vi "FL_Save_incrementally_ts.vi"(0 "Temporary file output path":path, 1 "Play / Pause":bool, 2 "Sensor read input":sgl[][](array[numeric]), 5 "Loop iteration":i32, 7 "Loop speed in ms":u16, 9 "Save every N seconds":u32=15, 11 "error in (no error)":errorcluster, 12 "Current_Time":timestamp, 13 "Start_Time":timestamp) -> (4 "Eff. save interval":sgl, 15 "error out":errorcluster)   [LabVIEW 2018, in "Tracker.lvlib"]
uses:
  Tracker.lvlib
  <vilib>/Utility/file.llb/Write Delimited Spreadsheet (DBL).vi
panel:
  out "transposed array":dbl[][](array[numeric])
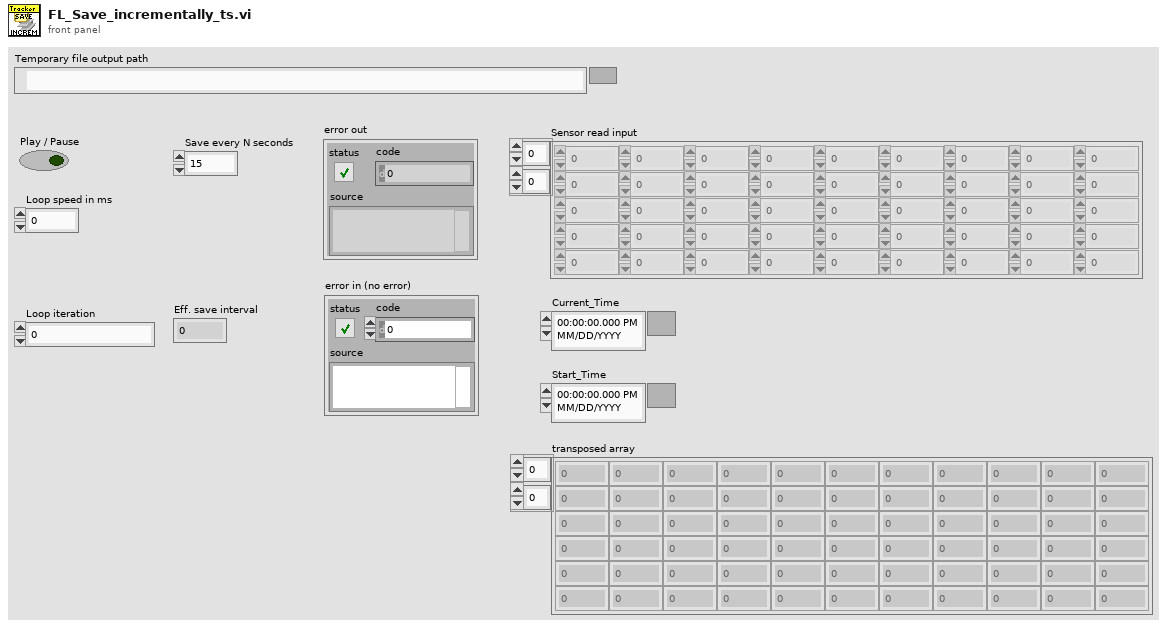
[diagram p1: front panel]
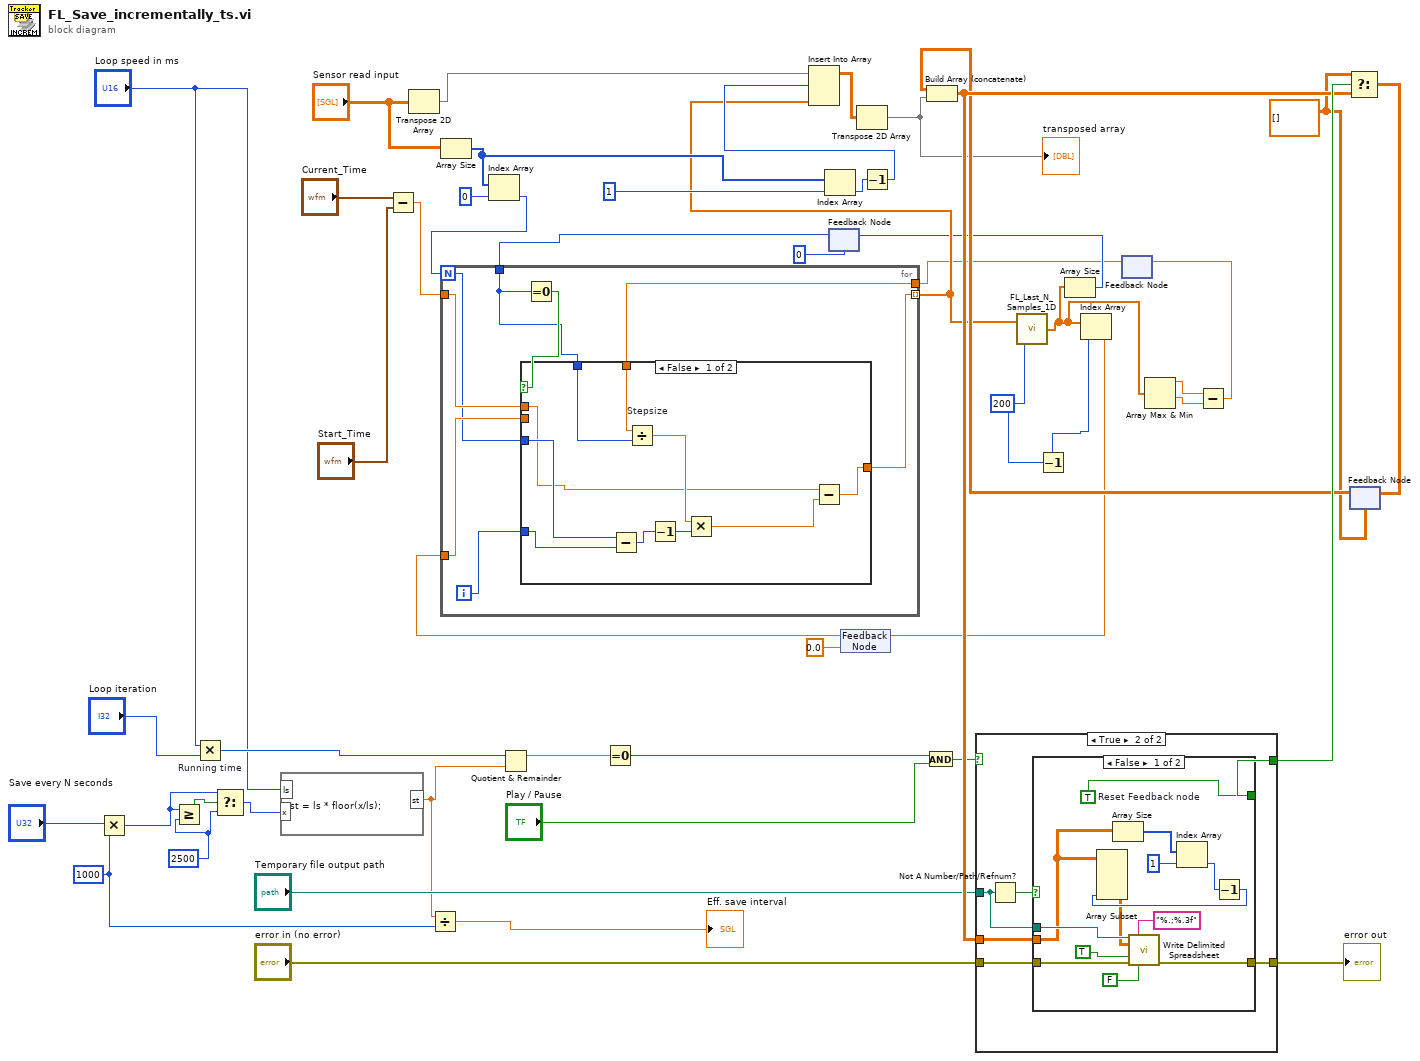
[diagram p0: block diagram]
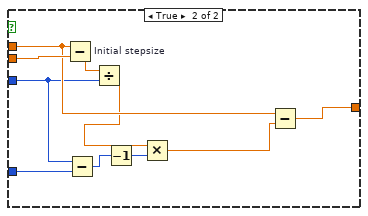
[diagram p2: hidden frame]
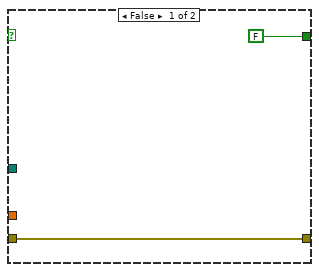
[diagram p3: hidden frame]
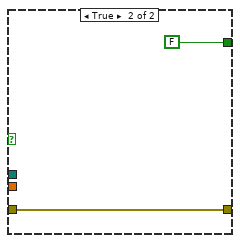
[diagram p4: hidden frame]
diagram:
  w13 = u32 200 ("BufferLengthSamples")
  w28 = u32 1000 ("y")
  w35 = 2500
  w39 = sgl[][] []
  n1 = Multiply(x="Save every N seconds", y=w28) -> (x*y=w31:u32)
  n2 = Greater Or Equal?(x=w31, y=w35) -> (x >= y?=w36:bool)
  n3 = Multiply "Running time"(x="Loop speed in ms", y="Loop iteration") -> (x*y=w42:i32)
  n4 = Select(t=w31, s=w36, f=w35) -> (s? t:f=w33:u32)
  n5 = formula code="st = ls * floor(x/ls);"("ls"="Loop speed in ms", "x"=w33) -> ("st"=w30:dbl)
  n6 = Subtract(x="Current_Time", y="Start_Time") -> (x-y=w22:dbl)
  n7 = Transpose 2D Array(2D array="Sensor read input") -> (transposed array=w21:sgl[][])
  n8 = Divide(x=w30, y=w28) -> (x/y=→"Eff. save interval":dbl)
  n9 = Array Size(array="Sensor read input") -> (size(s)=w19:i32[])
  n10 = Index Array(array=w19, index=0) -> (element=w15:i32)
  n11 = Quotient & Remainder(x=w42, y=w30) -> (x-y*floor(x/y)=w40:dbl)  [unwired: 1 out]
  n12 = Equal To 0?(x=w40) -> (x = 0?=w41:bool)
  n13 = Index Array(array=w19, index=1) -> (element=w17:i32)
  n14 = feedback #1(0) -> (w10:i32)
  n15 = feedback #2(sgl 0.0 ("SGL")) -> (w7:dbl)
  n16 = Decrement(x=w17) -> (x-1=w16:i32)
  n17 = And(x=w41, y="Play / Pause") -> (x .and. y?=w46:bool)
  n18 = Decrement(x=w13) -> (x-1=w12:u32)
  n19 = feedback #3() -> (w1:dbl)  [unwired: 1 in]
  n20 = for {
    N: w15 -> [w55]
    tunnel: w22 -> [w57]
    tunnel: [w54] -> w14 mode=indexing
    tunnel: w7 -> [w56]
    tunnel: w10 -> [w52]
    tunnel: w1 -> [w51]
    i -> [w53]
    n21 = Equal To 0?(x=w52) -> (x = 0?=w58:bool)
    n22 = case shown="False" w58 {
      tunnel: w57 -> [w60 w76]
      tunnel: w56 -> [_ w78]
      tunnel: w55 -> [w61 w72]
      tunnel: [w63 w75] -> w54
      tunnel: w53 -> [w62 w70]
      tunnel: w52 -> [w68 _]
      tunnel: w51 -> [w59 _]
      frame False {
        n23 = Subtract(x=w61, y=w62) -> (x-y=w66:i32)
        n24 = Divide "Stepsize"(x=w59, y=w68) -> (x/y=w64:dbl)
        n25 = Decrement(x=w66) -> (x-1=w65:i32)
        n26 = Multiply(x=w64, y=w65) -> (x*y=w67:dbl)
        n27 = Subtract(x=w60, y=w67) -> (x-y=w63:dbl)
      }
      frame True {
        n28 = Subtract(x=w76, y=w78) -> (x-y=w77:dbl)
        n29 = Subtract(x=w72, y=w70) -> (x-y=w71:i32)
        n30 = Divide "Initial stepsize"(x=w77, y=w72) -> (x/y=w74:dbl)
        n31 = Decrement(x=w71) -> (x-1=w69:i32)
        n32 = Multiply(x=w74, y=w69) -> (x*y=w73:dbl)
        n33 = Subtract(x=w76, y=w73) -> (x-y=w75:dbl)
      }
    }
  }
  n34 = Insert Into Array(array=w21, index (row)=w16, new element=w14) -> (w20:sgl[][])  [unwired: 1 in]
  n35 = Transpose 2D Array(2D array=w20) -> (transposed array=w27:sgl[][])
  "transposed array" <- w27
  n36 = call "FL_Last_N_Samples_1D.vi"("BufferLengthSamples"=w13, "Input Array"=w14) -> ("Output Array"=w5:dbl[])
  n37 = Array Size(array=w5) -> (size(s)=w11:i32)
  n38 = feedback-in #1(w11) -> ()
  n39 = Index Array(array=w5, index=w12) -> (element=w8:dbl)
  n40 = feedback-in #2(w8) -> ()
  n41 = Array Max & Min(array=w5) -> (max value=w4:dbl, min value=w3:dbl)  [unwired: 2 out]
  n42 = Subtract(x=w4, y=w3) -> (x-y=w2:dbl)
  n43 = feedback-in #3(w2) -> ()
  n44 = feedback #4(w39) -> (w47:sgl[][])
  n45 = Build Array (concatenate)(w47, w27) -> (w48:sgl[][])
  n46 = case shown="True" w46 {
    tunnel: "Temporary file output path" -> [_ w85]
    tunnel: w48 -> [_ w84]
    tunnel: [FALSE w83] -> w50
    tunnel: "error in (no error)" -> [w79 w82]
    tunnel: [w79 w81] -> w37
    frame False {
    }
    frame True {
      n47 = Not A Number/Path/Refnum?(number/path/refnum=w85) -> (NaN/Path/Refnum?=w86:bool)
      n48 = case shown="False" w86 {
        tunnel: w85 -> [w99 _]
        tunnel: w84 -> [w91 _]
        tunnel: [w96 FALSE] -> w83
        tunnel: w82 -> [w95 w100]
        tunnel: [w94 w100] -> w81
        frame False {
          w96 = TRUE  # Reset Feedback node
          n49 = Array Size(array=w91) -> (size(s)=w93:i32[])
          n50 = Index Array(array=w93, index=1) -> (element=w90:i32)
          n51 = Decrement(x=w90) -> (x-1=w89:i32)
          n52 = Array Subset(array=w91, length (col)=w89) -> (w88:sgl[][])  [unwired: 3 in]
          n53 = call-poly <vilib>:"Write Delimited Spreadsheet.vi"("file path (dialog if empty)"=w99, "format (%.3f)"="%.;%.3f", "2D data"=w88, "append to file? (new file:F)"=TRUE, "error in (no error)"=w95, "transpose? (no:F)"=FALSE) -> ("error out"=w94:errorcluster)  [unwired: 8 in, 1 out]
        }
        frame True {
        }
      }
    }
  }
  "error out" <- w37
  n54 = Select(t=w39, s=w50, f=w48) -> (s? t:f=w49:sgl[][])
  n55 = feedback-in #4(w49) -> ()
